vi "equalize_double_circ_trajectory.vi"(0 "TrajectoryTS090820Circular2D in":refnum<class "TrajectoryTS090820Circular2D.lvclass">, 5 "error in (no error)":errorcluster) -> (14 "TrajectoryTS090820Circular2D out":refnum<class "TrajectoryTS090820Circular2D.lvclass">, 15 "x trajectory":dbl[](array[numeric]), 16 "y trajectory":dbl[](array[numeric]), 17 "z trajectory":dbl[](array[numeric]), 18 "intensity":dbl[](array[numeric]), 19 "error out":errorcluster)   [LabVIEW 2010, in "TrajectoryTS090820Circular2D.lvclass"]
uses:
  TrajectoryTS090820Circular2D.lvclass
  <vilib>/Analysis/NI_AALBLAS.lvlib
  <vilib>/Analysis/BLAS.llb/dnrm2 - Vector 2-Norm (DBL).vi
panel:
  out "y trajectory":dbl[](graph)
  out "x trajectory":dbl[](graph)
  out "points AFTER equal-distribution":cluster{dbl, dbl}[](graph)
  out "loop counter":i32
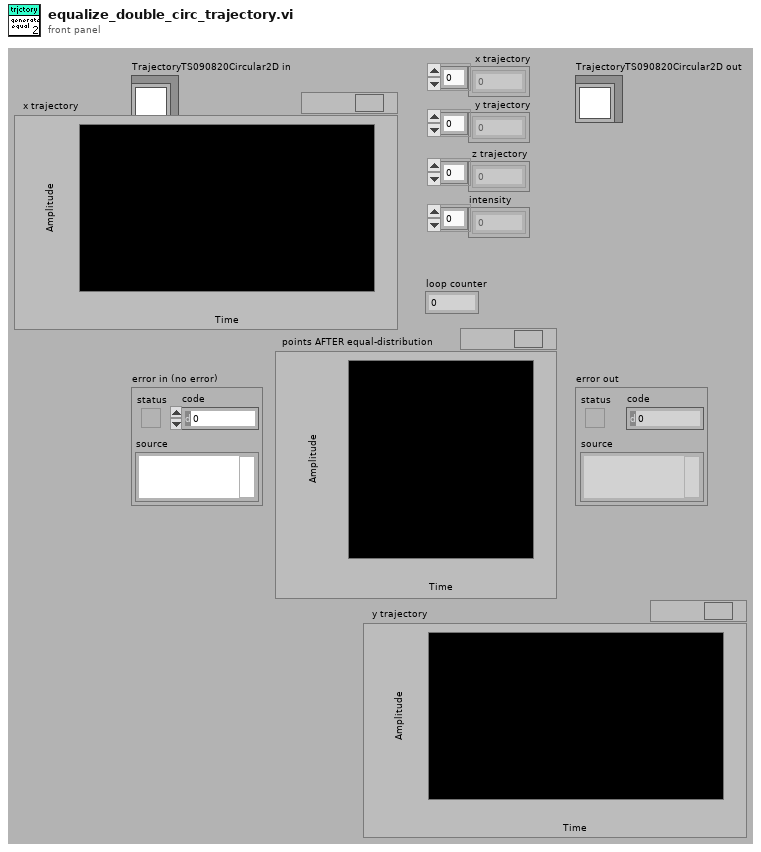
[diagram p1: front panel]
types:
  T1 = cluster{"total number of pixels per cycle":i32, "step":dbl, "x amplitude no units":dbl, "y amplitude no units":dbl, "x frequency":dbl, "y frequency ":dbl, "Phase shift":dbl}
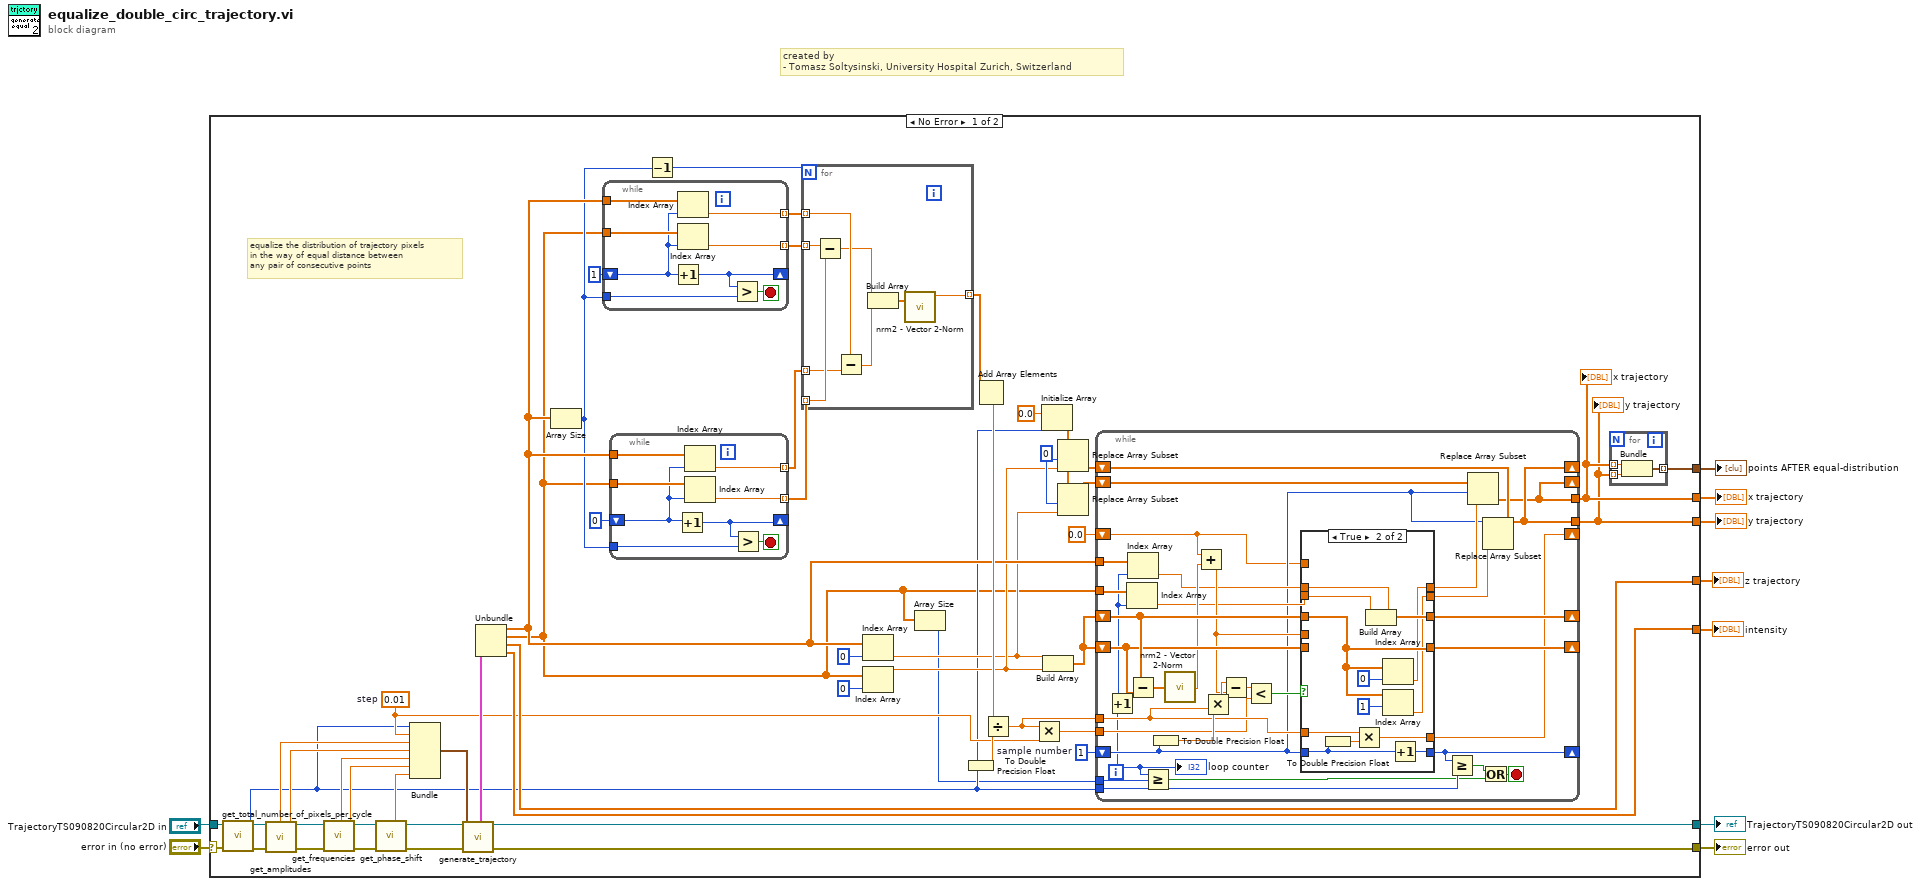
[diagram p0: block diagram]
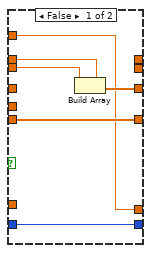
[diagram p2: hidden frame]
diagram:
  # "created by \n- Tomasz Soltysinski, University Hospital Zurich, Switzerland"
  n1 = case shown="No Error" "error in (no error)" {
    selector: "error in (no error)" -> [w61 w145]
    tunnel: [w33 w145] -> w8
    tunnel: [w34 w144] -> w6
    tunnel: "TrajectoryTS090820Circular2D in" -> [w62 w144]
    tunnel: [w20 _] -> w5
    tunnel: [w19 _] -> w4
    tunnel: [w23 _] -> w3
    tunnel: [w22 _] -> w2
    tunnel: [w21 _] -> w1
    frame No Error {
      w29 = 0 ("index")
      w14 = 0.01  # step
      w63 = 1  # sample number
      # "equalize the distribution of trajectory pixels \nin the way of equal distance between \nany pair of consecutive points"
      n2 = call-dynamic "get_total_number_of_pixels_per_cycle.vi"("error in (no error)"=w61, "TrajectoryTS090820Circular2D in"=w62) -> ("error out"=w46:errorcluster, "total number of pixels per cycle"=w12:i32, "TrajectoryTS090820Circular2D out"=w49:refnum<class "TrajectoryTS090820Circular2D.lvclass">)  [unwired: 7 in]
      n3 = call-dynamic "get_amplitudes.vi"("TrajectoryTS090820Circular2D in"=w49, "error in (no error)"=w46) -> ("TrajectoryTS090820Circular2D out"=w48:refnum<class "TrajectoryTS090820Circular2D.lvclass">, "x amplitude no units"=w43:dbl, "y amplitude no units"=w42:dbl, "error out"=w45:errorcluster)  [unwired: 12 in, 2 out]
      n4 = call-dynamic "get_frequencies.vi"("error in (no error)"=w45, "TrajectoryTS090820Circular2D in"=w48) -> ("error out"=w44:errorcluster, "y frequency"=w40:dbl, "x frequency"=w41:dbl, "TrajectoryTS090820Circular2D out"=w47:refnum<class "TrajectoryTS090820Circular2D.lvclass">)  [unwired: 6 in]
      n5 = call-dynamic "get_phase_shift.vi"("error in (no error)"=w44, "TrajectoryTS090820Circular2D in"=w47) -> ("error out"=w37:errorcluster, "Phase shift"=w39:dbl, "TrajectoryTS090820Circular2D out"=w38:refnum<class "TrajectoryTS090820Circular2D.lvclass">)  [unwired: 7 in]
      n6 = Bundle("total number of pixels per cycle"=w12, "step"=w14, "x amplitude no units"=w43, "y amplitude no units"=w42, "x frequency"=w41, "y frequency"=w40, "Phase shift"=w39) -> (w35:T1)  [unwired: 1 in]
      n7 = call-dynamic "generate_trajectory.vi"("TrajectoryTS090820Circular2D in"=w38, "trajectory params"=w35, "error in (no error)"=w37) -> ("TrajectoryTS090820Circular2D out"=w34:refnum<class "TrajectoryTS090820Circular2D.lvclass">, "trajectory"=w28:cluster{dbl[], dbl[], dbl[], dbl[]}, "error out"=w33:errorcluster)  [unwired: 14 in]
      n8 = Unbundle(w28) -> (w27:dbl[], w11:dbl[], w22:dbl[], w21:dbl[])
      n9 = Array Size(array=w27) -> (size(s)=w25:i32)
      n10 = while {
        shift-right: [w83] -> _
        shift-left: 1 -> [w84]
        tunnel: w11 -> [w85]
        tunnel: [w90] -> w55 mode=indexing
        tunnel: w27 -> [w89]
        tunnel: [w88] -> w26 mode=indexing
        tunnel: w25 -> [w87]
        stop <- w86 stop-if-true
        n11 = Increment(x=w84) -> (x+1=w83:i32)
        n12 = Index Array(array=w89, index=w84) -> (element=w88:dbl)
        n13 = Index Array(array=w85, index=w84) -> (element=w90:dbl)
        n14 = Greater?(x=w83, y=w87) -> (0:w86:bool)
      }
      n15 = while {
        tunnel: w11 -> [w77]
        shift-right: [w75] -> _
        shift-left: 0 -> [w76]
        tunnel: [w82] -> w54 mode=indexing
        tunnel: w27 -> [w81]
        tunnel: [w80] -> w53 mode=indexing
        tunnel: w25 -> [w79]
        stop <- w78 stop-if-true
        n16 = Increment(x=w76) -> (x+1=w75:i32)
        n17 = Index Array(array=w81, index=w76) -> (element=w80:dbl)
        n18 = Index Array(array=w77, index=w76) -> (element=w82:dbl)
        n19 = Greater?(x=w75, y=w79) -> (0:w78:bool)
      }
      n20 = Decrement(x=w25) -> (x-1=w24:i32)
      n21 = for {
        N: w24 -> [_]
        tunnel: w55 -> [w74] mode=indexing
        tunnel: w54 -> [w73] mode=indexing
        tunnel: w53 -> [w72] mode=indexing
        tunnel: w26 -> [w71] mode=indexing
        tunnel: [w67] -> w52 mode=indexing
        n22 = Subtract(x=w74, y=w73) -> (x-y=w69:dbl)
        n23 = Subtract(x=w71, y=w72) -> (x-y=w70:dbl)
        n24 = Build Array(w69, w70) -> (w68:dbl[])
        n25 = call-poly <vilib>:"nrm2 - Vector 2-Norm.vi"("x"=w68) -> ("dnrm2"=w67:dbl)  [unwired: 9 in, 1 out]
      }
      n26 = Index Array(array=w27, index=0) -> (element=w17:dbl)
      n27 = Index Array(array=w11, index=0) -> (element=w18:dbl)
      n28 = Array Size(array=w11) -> (size(s)=w10:i32)
      n29 = To Double Precision Float(number=w12) -> (double precision float=w51:dbl)
      n30 = Add Array Elements(numeric array=w52) -> (sum=w50:dbl)
      n31 = Divide(x=w50, y=w51) -> (x/y=w13:dbl)
      n32 = Multiply(x=w13, y=w14) -> (x*y=w15:dbl)
      n33 = Initialize Array(0.0, w12) -> (w30:dbl[])
      n34 = Build Array(w17, w18) -> (w36:dbl[])
      n35 = Replace Array Subset(array=w30, new element=w18, index=w29) -> (w32:dbl[])
      n36 = Replace Array Subset(array=w30, new element=w17, index=w29) -> (w31:dbl[])
      n37 = while {
        tunnel: w12 -> [w124]
        shift-right: [w117] -> _
        shift-left: w63 -> [w98]
        tunnel: w15 -> [w103]
        shift-right: [w123] -> _
        shift-left: w36 -> [w121]
        shift-right: [w122] -> _
        shift-left: w36 -> [w120]
        tunnel: [w111] -> w20
        tunnel: [w112] -> w19
        shift-right: [w112] -> _
        shift-left: w32 -> [w114]
        shift-right: [w111] -> _
        shift-left: w31 -> [w113]
        tunnel: w27 -> [w102]
        tunnel: w11 -> [w100]
        shift-right: [w110] -> _
        shift-left: 0.0 -> [w96]
        tunnel: w13 -> [w108]
        tunnel: w10 -> [w95]
        i -> [w94]
        stop <- w91 stop-if-true
        n38 = Increment(x=w94) -> (x+1=w97:i32)
        n39 = Index Array(array=w100, index=w97) -> (element=w99:dbl)
        n40 = Index Array(array=w102, index=w97) -> (element=w101:dbl)
        n41 = Subtract(x=w121, y=w120) -> (x-y=w119:dbl[])
        n42 = Greater Or Equal?(x=w94, y=w95) -> (x >= y?=w92:bool)
        n43 = To Double Precision Float(number=w98) -> (double precision float=w109:dbl)
        n44 = call-poly <vilib>:"nrm2 - Vector 2-Norm.vi"("x"=w119) -> ("dnrm2"=w107:dbl)  [unwired: 9 in, 1 out]
        n45 = Add(x=w96, y=w107) -> (x+y=w105:dbl)
        n46 = Multiply(x=w108, y=w109) -> (x*y=w106:dbl)
        n47 = Subtract(x=w106, y=w105) -> (x-y=w104:dbl)
        n48 = Less?(x=w104, y=w103) -> (x < y?=w118:bool)
        n49 = case shown="True" w118 {
          tunnel: w98 -> [w130 w141]
          tunnel: [w130 w143] -> w117
          tunnel: [w128 w142] -> w123
          tunnel: w121 -> [_ w135]
          tunnel: w120 -> [w129 _]
          tunnel: [w129 w135] -> w122
          tunnel: w101 -> [w127 w134]
          tunnel: w99 -> [w126 w132]
          tunnel: [_ w133] -> w116
          tunnel: [_ w131] -> w115
          tunnel: w108 -> [_ w139]
          tunnel: [w125 w138] -> w110
          tunnel: w105 -> [_ _]
          tunnel: w96 -> [w125 _]
          frame False {
            n50 = Build Array(w127, w126) -> (w128:dbl[])
          }
          frame True {
            n51 = To Double Precision Float(number=w141) -> (double precision float=w140:dbl)
            n52 = Multiply(x=w139, y=w140) -> (x*y=w138:dbl)
            n53 = Build Array(w134, w132) -> (w142:dbl[])
            n54 = Index Array(array=w135, index=0) -> (element=w133:dbl)
            n55 = Index Array(array=w135, index=1) -> (element=w131:dbl)
            n56 = Increment(x=w141) -> (x+1=w143:i32)
          }
        }
        n57 = Greater Or Equal?(x=w117, y=w124) -> (x >= y?=w93:bool)
        n58 = Replace Array Subset(array=w113, new element=w116, index=w98) -> (w111:dbl[])
        n59 = Or(x=w93, y=w92) -> (x .or. y?=w91:bool)
        n60 = Replace Array Subset(array=w114, new element=w115, index=w98) -> (w112:dbl[])
        "loop counter" <- w94
      }
      "x trajectory" <- w20
      "y trajectory" <- w19
      n61 = for {
        tunnel: [w66] -> w23 mode=indexing
        tunnel: w20 -> [w65] mode=indexing
        tunnel: w19 -> [w64] mode=indexing
        n62 = Bundle(w65, w64) -> (w66:cluster{dbl, dbl})  [unwired: 1 in]
      }
    }
    frame Error {
    }
  }
  "error out" <- w8
  "TrajectoryTS090820Circular2D out" <- w6
  "x trajectory" <- w5
  "y trajectory" <- w4
  "points AFTER equal-distribution" <- w3
  "z trajectory" <- w2
  "intensity" <- w1
